vi "Frame Clock.vi"(0 "Start of Frame":bool, 1 "End of Frame":bool, 2 "Reset":bool) -> (6 "Frame Clock Out":bool)   [LabVIEW 2014]
panel:
  # "Copyright 2014 Vidrio Technologies\nScanImage 5 software is licensed under the Apache License, Version 2.0 (the \"License\"); you may not use any files contained\nwithin the ScanImage 5 release except in compliance with the License. You may obtain a copy of the License at\n http://www.apache.org/licenses/LICENSE-2.0\nUnless required by applicable law or agreed to in writing, software distributed under the License is distributed on an\n\"AS IS\" BASIS, WITHOUT WARRANTIES OR CONDITIONS OF ANY KIND, either express or implied. See the License for the\n specific language governing permissions and limitations under the License."
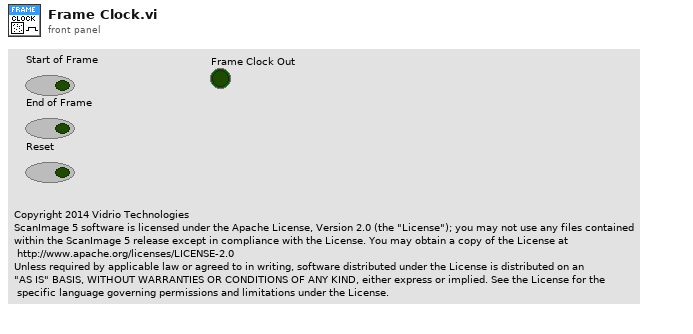
[diagram p1: front panel]
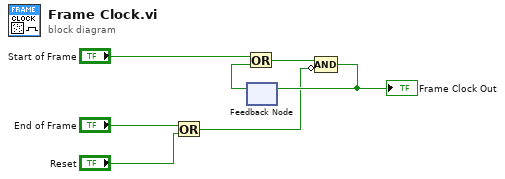
[diagram p0: block diagram]
diagram:
  n1 = Or(x="End of Frame", y="Reset") -> (x .or. y?=w1:bool)
  n2 = feedback #1() -> (w5:bool)  [unwired: 1 in]
  n3 = Or(x="Start of Frame", y=w5) -> (x .or. y?=w7:bool)
  n4 = Compound Arithmetic op=AND(w7, invert w1) -> (w6:bool)
  "Frame Clock Out" <- w6
  n5 = feedback-in #1(w6) -> ()
